vi "GOOP_GetProviderIniFilePath.vi"() -> (1 "ProviderMainFolder":path, 2 "ProviderIniPath":path)   [LabVIEW 2020]
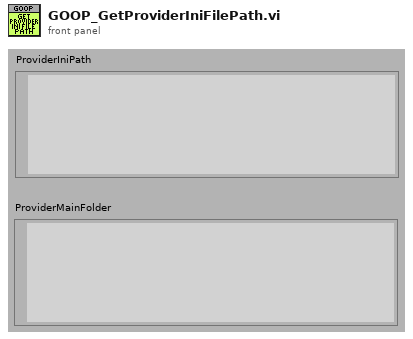
[diagram p1: front panel]
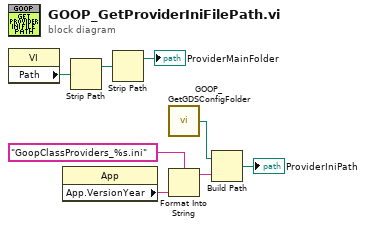
[diagram p0: block diagram]
diagram:
  n1 = property class="VI"() -> ("Path"=w8:path)  [unwired: 2 in, 2 out]
  n2 = property class="App"() -> ("App.VersionYear"=w3:string)  [unwired: 2 in, 2 out]
  n3 = Strip Path(path=w8) -> (stripped path=w7:path)  [unwired: 1 out]
  n4 = Strip Path(path=w7) -> (stripped path=→"ProviderMainFolder":path)  [unwired: 1 out]
  n5 = call <resource>:"GOOP_GetGDSConfigFolder.vi"() -> ("GDSFolderPath"=w4:path)
  n6 = Format Into String(format string="GoopClassProviders_%s.ini" ("name or relative path"), w3) -> (resulting string=w1:string)  [unwired: 2 in, 1 out]
  n7 = Build Path(base path=w4, name or relative path=w1) -> (appended path=→"ProviderIniPath":path)
